vi "Clean Up Actor.vi"(8 "error in (no error)":errorcluster, 11 "Bank Account in":refnum<class "Bank Account.lvclass">) -> (0 "error out":errorcluster, 3 "Bank Account out":refnum<class "Bank Account.lvclass">)   [LabVIEW 2016, in "CLD Exam - ATM.lvlib" / "Bank Account.lvclass"]
uses:
  Bank Account.lvclass
  D:/Repos/Stream/software/Mediator/Classes/Mediated Actor/Mediated Actor.lvclass
  Mediator/Classes/Message Broker Interface/Message Broker Interface.lvclass
  Mediator/Classes/Mediated Synchronous Actor/Mediated Synchronous Actor.lvclass
  Mediator/Classes/Mediated Actor/Mediated Actor.lvclass
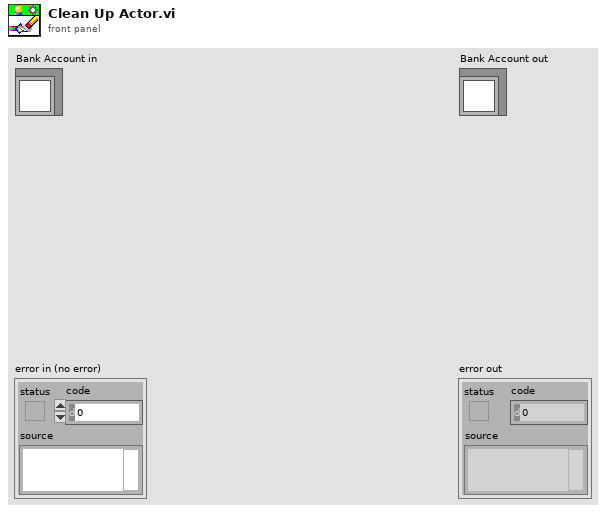
[diagram p1: front panel]
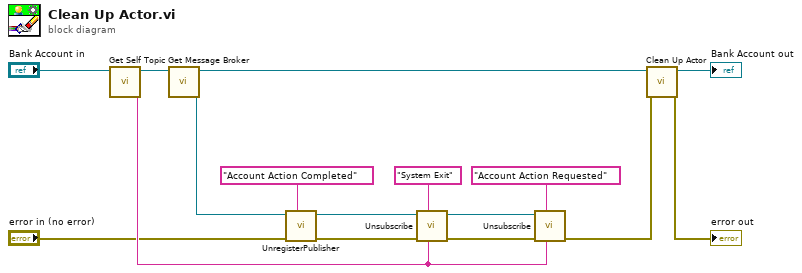
[diagram p0: block diagram]
diagram:
  n1 = call "Get Self Topic.vi"("Mediated Actor in"="Bank Account in") -> ("Topic.Self"=w7:string, "Mediated Actor out"=w12:refnum<class "Bank Account.lvclass">)  [unwired: 9 in]
  n2 = call "Get Message Broker.vi"("Mediated Actor in"=w12) -> ("Message Broker"=w6:refnum<class "Message Broker Interface.lvclass">, "Mediated Actor out"=w10:refnum<class "Bank Account.lvclass">)  [unwired: 9 in]
  n3 = call-dynamic "UnregisterPublisher.vi"("Topic Name"="Account Action Completed", "error in (no error)"="error in (no error)", "Message Broker Interface in"=w6) -> ("error out"=w3:errorcluster, "Message Broker Interface out"=w4:refnum<class "Message Broker Interface.lvclass">)  [unwired: 7 in]
  n4 = call-dynamic "Unsubscribe.vi"("Subscriber Name"=w7, "Topic Name"="System Exit", "error in (no error)"=w3, "Message Broker Interface in"=w4) -> ("error out"=w1:errorcluster, "Message Broker Interface out"=w2:refnum<class "Message Broker Interface.lvclass">)  [unwired: 6 in]
  n5 = call-dynamic "Unsubscribe.vi"("Subscriber Name"=w7, "Topic Name"="Account Action Requested", "error in (no error)"=w1, "Message Broker Interface in"=w2) -> ("error out"=w8:errorcluster)  [unwired: 6 in, 1 out]
  n6 = call-parent "Clean Up Actor.vi"("error in (no error)"=w8, "Mediated Actor in"=w10) -> ("error out"=→"error out":errorcluster, "Mediated Actor out"=→"Bank Account out":refnum<class "Bank Account.lvclass">)  [unwired: 8 in]
